vi "get db wheel info.vi"() -> ()   [LabVIEW 2016]
uses:
  <vilib>/addons/database/Connection.llb/DB Tools Open Connec (String).vi
  <vilib>/addons/database/Connection.llb/Conn Execute.vi
  <vilib>/addons/database/Recordset.llb/Rec Fetch Recordset Data (R).vi
  <vilib>/addons/database/Recordset.llb/Rec Destroy - Connection.vi
  <vilib>/Utility/file.llb/Write Delimited Spreadsheet (string).vi
  <vilib>/addons/database/NI_Database_API.lvlib
panel:
  out "size(s)":i32
  out "data":timestamp[](array[timestamp])
  out "date/time string 2":string
  out "date/time string":string
  out "sorted array":timestamp[](array[timestamp])
  out "element":string
  out "output array":string[][](array[string])
  out "Array 3":string[](array[string])
  out "Numeric":i32
  out "Array 4":string[](array[string])
  out "subarray":string[](array[string])
  out "Array 2":i16[](array[numeric])
  out "qa per group":dbl
  out "blanks per group":dbl
  out "unknown per group":dbl
  out "number of groups":dbl
  out "unknowns":i32
  out "qa number of":i32
  out "blanks number of":i32
  out "standards number of":i32
  out "x-y":dbl[](array[numeric])
  out "recordset data 2":variant[][](array[variant])
  out "concatenated string":string
  in  "wheel number":dbl=1.0
  out "error out 2":errorcluster
  in  "Ring":u16(ring)=1 items=["10Be"=1, "14C"=2, "26Al"=3, "36Cl"=5, "41Ca"=6, "129I"=7]
  out "Array":string[](array[string])
  out "error out":errorcluster
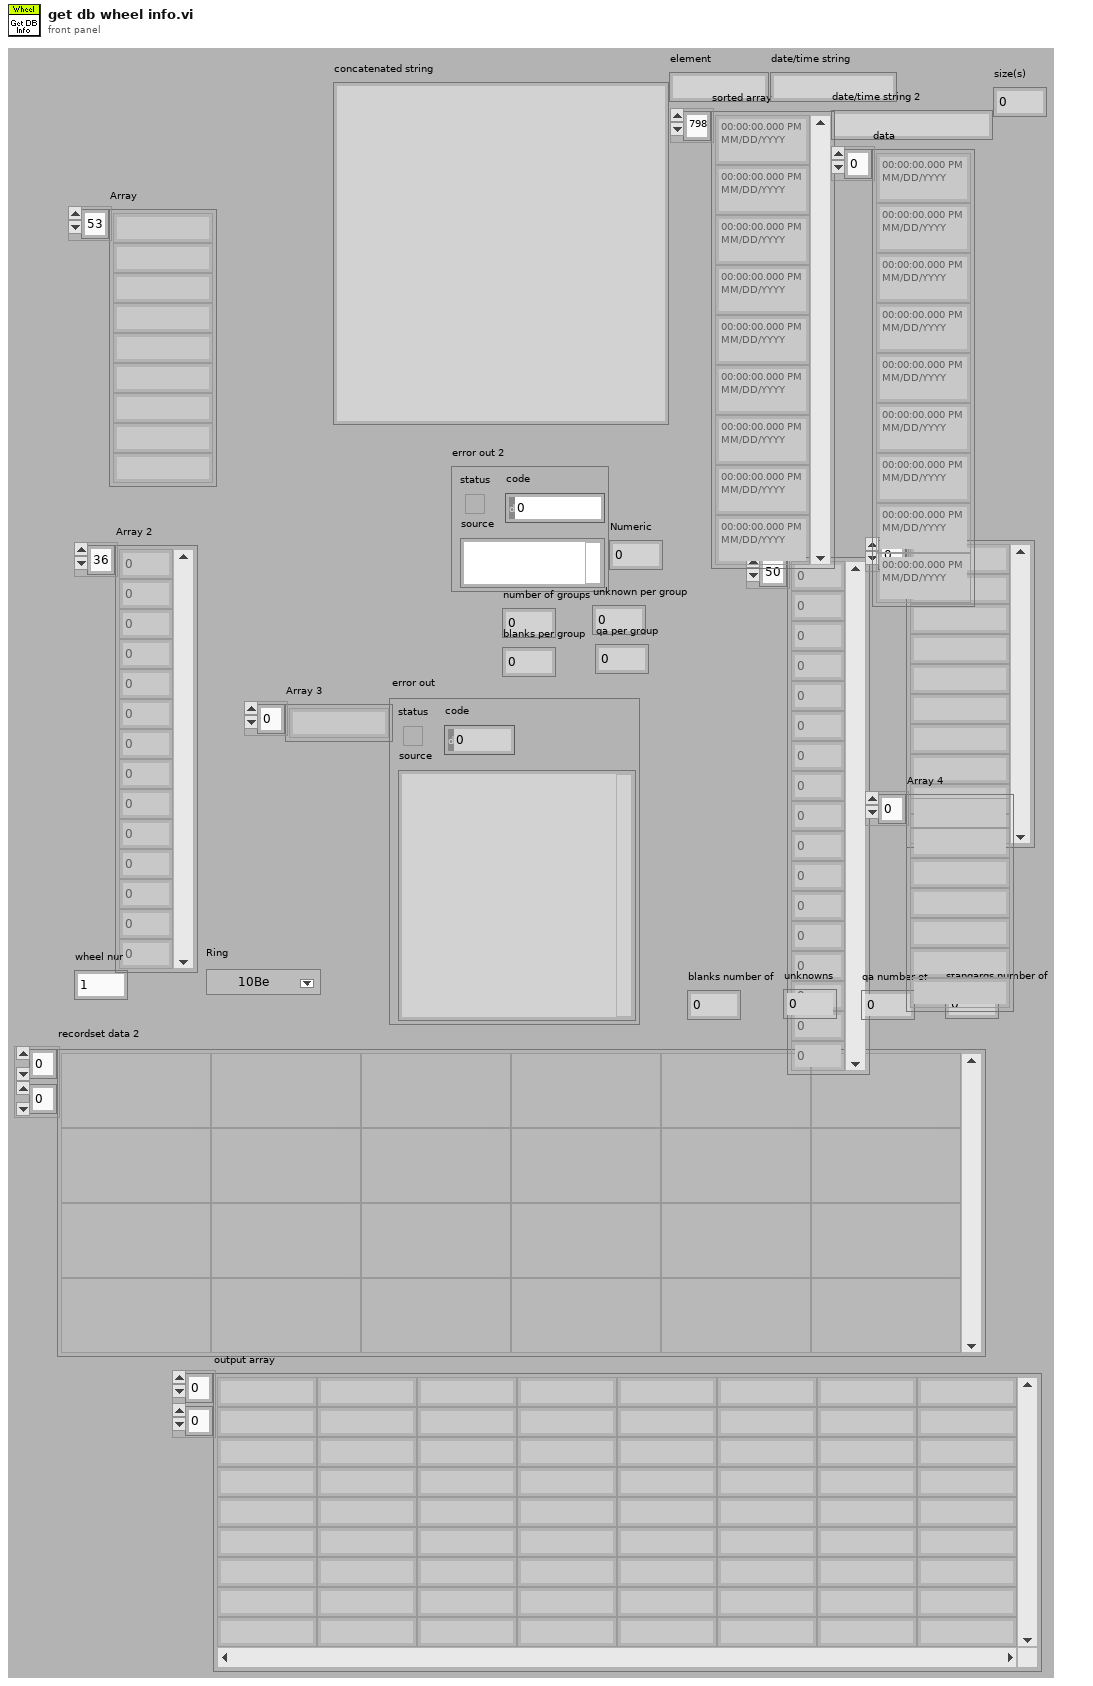
[diagram p1: front panel]
types:
  T1 = typedef "NI_Database_API.lvlib/Conn ObjectReference.ctl" = refnum<k1>
  T2 = typedef "NI_Database_API.lvlib/Rec ObjectReference.ctl" = refnum<k1>
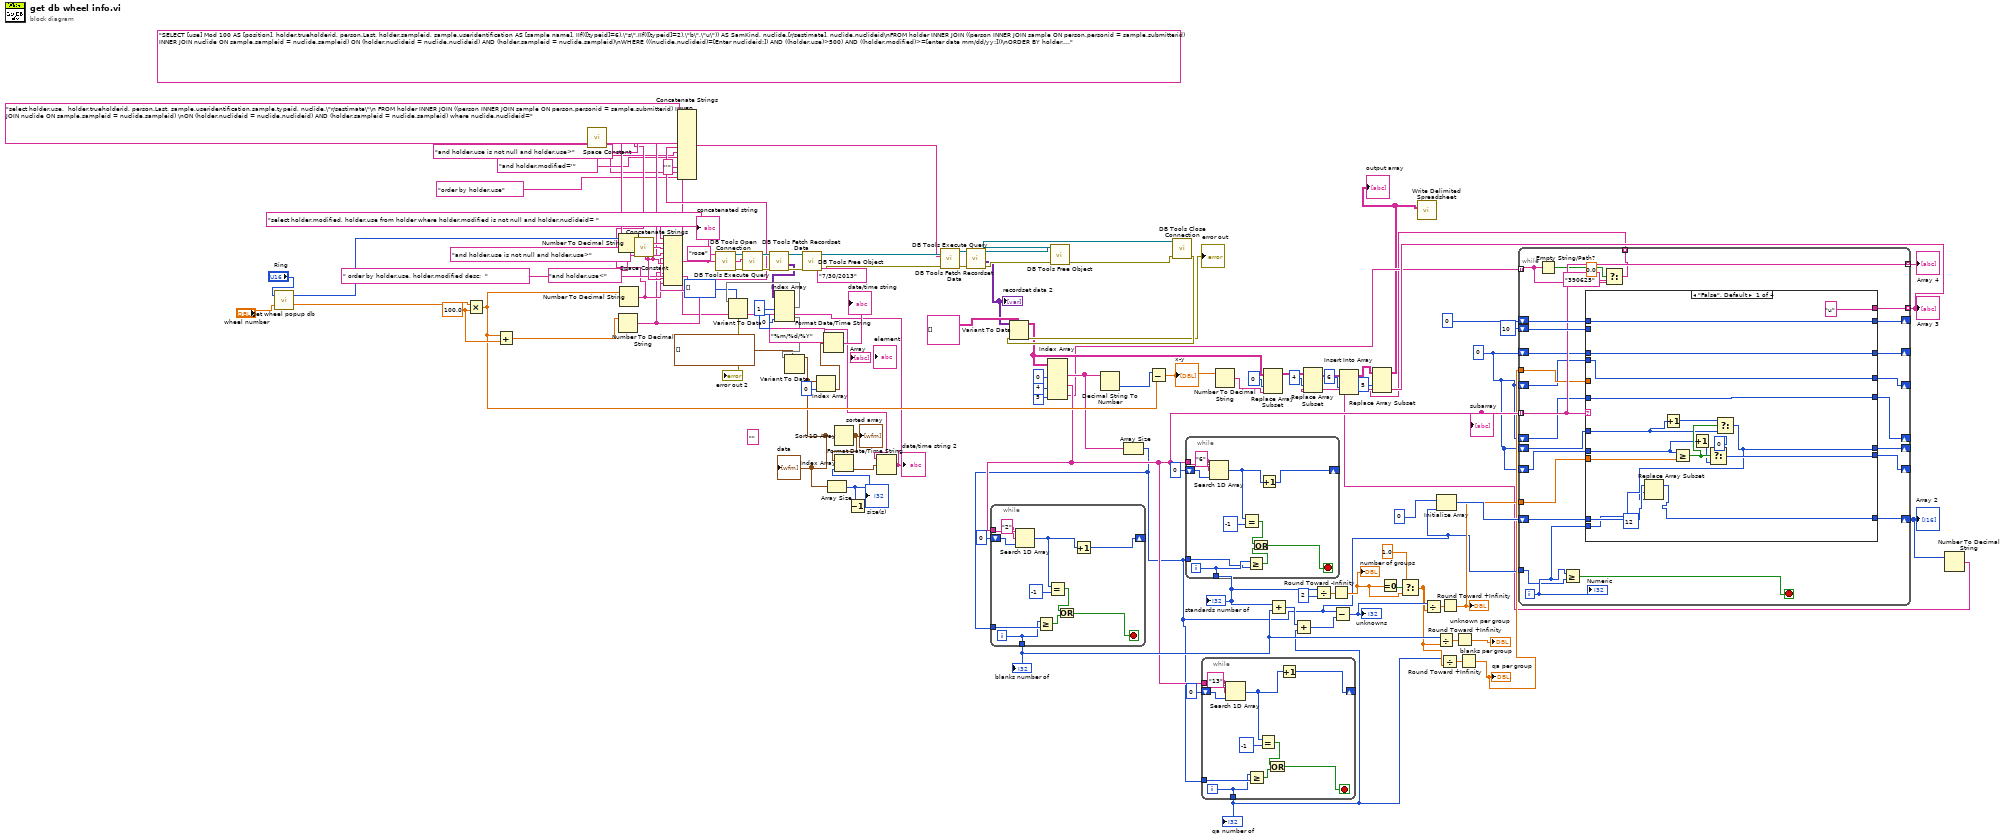
[diagram p0: block diagram]
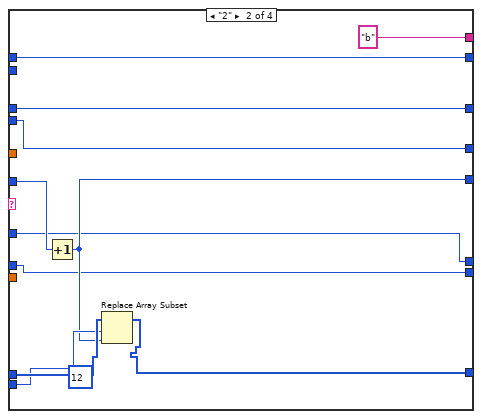
[diagram p2: hidden frame]
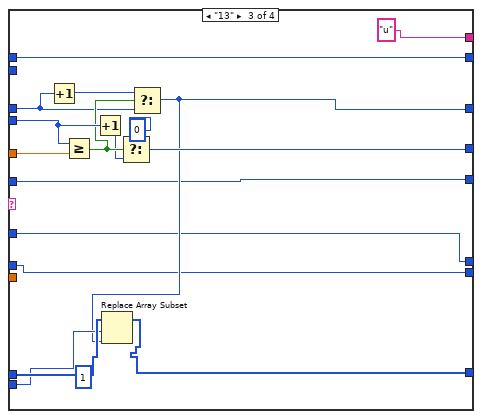
[diagram p3: hidden frame]
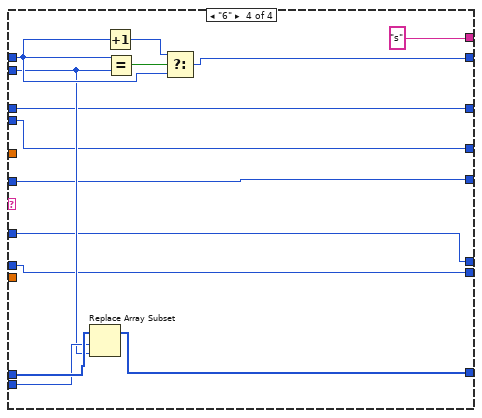
[diagram p4: hidden frame]
diagram:
  w6 = "%m/%d/%Y" ("time format string (%c)")
  (unwired) ""
  (unwired) "7/30/2013" ("element")
  w30 = i8 0 ("t")
  (unwired) "SELECT [use] Mod 100 AS [position], holder.trueholderid, person.Last, holder.sampleid, sample.useridentification AS [sample name], IIf(([typeid]=6),\"s\",IIf(([typeid]=2),\"b\",\"u\")) AS SamKind, nuclide.[r/sestimate], nuclide.nuclideid\nFROM holder INNER JOIN ((person INNER JOIN sample ON person.personid = sample.submitterid) INNER JOIN nuclide ON sample.sampleid = nuclide.sampleid) ON (holder.nuclideid = nuclide.nuclideid) AND (holder.sampleid = nuclide.sampleid)\nWHERE (((nuclide.nuclideid)=[Enter nuclideid:]) AND ((holder.use)>500) AND ((holder.modified)>=[enter date mm/dd/yy:]))\nORDER BY holder.use, [use] Mod 100" ("SQL query")
  w74 = "and holder.use<" ("SQL query")
  w90 = 100.0 ("y")
  n1 = call "get wheel popup db.vi"("wheel number"="wheel number", "Ring"="Ring") -> ("wheel number 2"=w91:dbl, "Ring 2"=w95:u16)
  n2 = Multiply(x=w91, y=w90) -> (x*y=w59:dbl)
  n3 = Add(x=w59, y=w90) -> (x+y=w89:dbl)
  n4 = call <vilib>:"Space Constant.vi"() -> ("String"=w69:string)
  n5 = Number To Decimal String(number=w89) -> (decimal integer string=w73:string)  [unwired: 1 in]
  n6 = Number To Decimal String(number=w95) -> (decimal integer string=w77:string)  [unwired: 1 in]
  n7 = Number To Decimal String(number=w59) -> (decimal integer string=w75:string)  [unwired: 1 in]
  n8 = call <vilib>:"Space Constant.vi"() -> ("String"=w88:string)
  n9 = Concatenate Strings("select holder.modified, holder.use from holder where holder.modified is not null and holder.nuclideid= " ("SQL query"), w77, w88, "and holder.use is not null and holder.use>" ("SQL query"), w75, w88, w74, w73, w88, " order by holder.use, holder.modified desc;  " ("SQL query")) -> (w94:string)
  "concatenated string" <- w94
  n10 = call-poly <vilib>:"DB Tools Open Connection.vi"("connection information"="rose") -> ("error out"=w104:errorcluster, "connection reference"=w105:T1)  [unwired: 7 in]
  n11 = call-poly <vilib>:"DB Tools Execute Query.vi"("error in (no error)"=w104, "SQL query"=w94, "connection reference"=w105) -> ("error out"=w108:errorcluster, "recordset reference"=w107:T2)  [unwired: 5 in]
  n12 = call-poly <vilib>:"DB Tools Fetch Recordset Data.vi"("error in (no error)"=w108, "recordset reference"=w107) -> ("error out"=w110:errorcluster, "recordset data"=w92:variant[][], "recordset reference out"=w109:T2)  [unwired: 3 in]
  n13 = Index Array(array=w92, index (col) #1=1 ("disabled index (col)"), index (col) #2=0 ("index (col)")) -> (element #1=w102:variant[], element #2=w99:variant[])  [unwired: 2 in]
  n14 = Variant To Data(type=i32[] [], Variant=w102) -> (error out=→"error out 2":errorcluster)  [unwired: 1 in, 1 out]
  n15 = Variant To Data(type=timestamp[] [], Variant=w99) -> (data=w9:timestamp[])  [unwired: 1 in, 1 out]
  "data" <- w9
  n16 = call-poly <vilib>:"DB Tools Free Object.vi"("error in (no error)"=w110, "recordset reference"=w109) -> ("error out"=w85:errorcluster, "connection reference"=w84:T1)  [unwired: 8 in]
  n17 = Index Array(array=w9, index=0) -> (element=w11:timestamp)
  n18 = Format Date/Time String(time format string (%c)=w6, seconds (now)=w11) -> (date/time string=→"date/time string":string)  [unwired: 1 in]
  n19 = Array Size(array=w9) -> (size(s)=w7:i32)
  "size(s)" <- w7
  n20 = Sort 1D Array(array=w9) -> (sorted array=w3:timestamp[])
  "sorted array" <- w3
  n21 = Decrement(x=w7) -> (x-1=w4:i32)
  n22 = Index Array(array=w3, index=w4) -> (element=w8:timestamp)
  n23 = Format Date/Time String(time format string (%c)=w6, seconds (now)=w8) -> (date/time string=w2:string)  [unwired: 1 in]
  "date/time string 2" <- w2
  n24 = Concatenate Strings("select holder.use,  holder.trueholderid, person.Last, sample.useridentification,sample.typeid, nuclide.\"r/sestimate\"\n FROM holder INNER JOIN ((person INNER JOIN sample ON person.personid = sample.submitterid) INNER JOIN nuclide ON sample.sampleid = nuclide.sampleid) \nON (holder.nuclideid = nuclide.nuclideid) AND (holder.sampleid = nuclide.sampleid) where nuclide.nuclideid=" ("SQL query"), w77, w69, "and holder.use is not null and holder.use>" ("SQL query"), w75, w69, w74, w73, w69, "and holder.modified='" ("string"), w2, "'" ("string"), w69, "order by holder.use" ("string")) -> (w72:string)
  n25 = call-poly <vilib>:"DB Tools Execute Query.vi"("error in (no error)"=w85, "SQL query"=w72, "connection reference"=w84) -> ("error out"=w79:errorcluster, "recordset reference"=w86:T2)  [unwired: 5 in]
  n26 = call-poly <vilib>:"DB Tools Fetch Recordset Data.vi"("error in (no error)"=w79, "recordset reference"=w86) -> ("error out"=w83:errorcluster, "recordset data"=w66:variant[][], "recordset reference out"=w82:T2)  [unwired: 3 in]
  "recordset data 2" <- w66
  n27 = call-poly <vilib>:"DB Tools Free Object.vi"("error in (no error)"=w83, "recordset reference"=w82) -> ("error out"=w80:errorcluster, "connection reference"=w81:T1)  [unwired: 8 in]
  n28 = call <vilib>:"DB Tools Close Connection.vi"("error in (no error)"=w80, "connection reference"=w81) -> ("error out"=w65:errorcluster)  [unwired: 5 in]
  n29 = Variant To Data(error in=w65, type=string[][] [], Variant=w66) -> (data=w28:string[][], error out=→"error out":errorcluster)
  n30 = Index Array(array=w28, index (col) #1=0 ("disabled index (col)"), index (col) #2=4 ("index (col)"), index (col) #3=5 ("index (col)")) -> (element #1=w58:string[], element #2=w38:string[], element #3=w15:string[])  [unwired: 3 in]
  "subarray" <- w38
  n31 = Decimal String To Number(string=w58) -> (number=w60:i32[])  [unwired: 2 in, 1 out]
  n32 = Array Size(array=w58) -> (size(s)=w26:i32)
  n33 = while {
    tunnel: w38 -> [w121]
    shift-right: [w111] -> _
    shift-left: 0 ("index of element") -> [w119]
    tunnel: w26 -> [w116]
    tunnel: [w113] -> w44
    i -> [w113]
    stop <- w114 stop-if-true
    n34 = Search 1D Array(1D array=w121, element="2", start index (0)=w119) -> (index of element=w112:i32)
    n35 = Greater Or Equal?(x=w113, y=w116) -> (x >= y?=w115:bool)
    n36 = Equal?(x=w112, y=-1) -> (x = y?=w117:bool)
    n37 = Or(x=w117, y=w115) -> (x .or. y?=w114:bool)
    n38 = Increment(x=w112) -> (x+1=w111:i32)
  }
  "blanks number of" <- w44
  n39 = Subtract(x=w60, y=w59) -> (x-y=w29:dbl[])
  "x-y" <- w29
  n40 = while {
    tunnel: w38 -> [w132]
    shift-right: [w125] -> _
    shift-left: 0 ("index of element") -> [w130]
    tunnel: w26 -> [w122]
    tunnel: [w123] -> w52
    i -> [w123]
    stop <- w127 stop-if-true
    n41 = Search 1D Array(1D array=w132, element="6", start index (0)=w130) -> (index of element=w126:i32)
    n42 = Equal?(x=w126, y=-1) -> (x = y?=w128:bool)
    n43 = Greater Or Equal?(x=w123, y=w122) -> (x >= y?=w124:bool)
    n44 = Or(x=w128, y=w124) -> (x .or. y?=w127:bool)
    n45 = Increment(x=w126) -> (x+1=w125:i32)
  }
  "standards number of" <- w52
  n46 = while {
    tunnel: w38 -> [w143]
    shift-right: [w133] -> _
    shift-left: 0 ("index of element") -> [w141]
    tunnel: w26 -> [w138]
    tunnel: [w135] -> w39
    i -> [w135]
    stop <- w136 stop-if-true
    n47 = Search 1D Array(1D array=w143, element="13", start index (0)=w141) -> (index of element=w134:i32)
    n48 = Greater Or Equal?(x=w135, y=w138) -> (x >= y?=w137:bool)
    n49 = Equal?(x=w134, y=-1) -> (x = y?=w139:bool)
    n50 = Or(x=w139, y=w137) -> (x .or. y?=w136:bool)
    n51 = Increment(x=w134) -> (x+1=w133:i32)
  }
  "qa number of" <- w39
  n52 = Number To Decimal String(number=w29) -> (decimal integer string=w27:string[])  [unwired: 1 in]
  n53 = Replace Array Subset(array=w28, new element=w27, index (col)=0 ("disabled index (col)")) -> (w25:string[][])  [unwired: 1 in]
  n54 = Add(x=w52, y=w44) -> (x+y=w54:i32)
  n55 = Add(x=w54, y=w39) -> (x+y=w53:i32)
  n56 = Divide(x=w52, y=2) -> (x/y=w50:dbl)
  n57 = Round Toward -Infinity(1:w50) -> (0:w47:dbl)
  "number of groups" <- w47
  n58 = Subtract(x=w26, y=w53) -> (x-y=w46:i32)
  "unknowns" <- w46
  n59 = Equal To 0?(x=w47) -> (x = 0?=w49:bool)
  n60 = Select(t=1.0, s=w49, f=w47) -> (s? t:f=w43:dbl)
  n61 = Divide(x=w46, y=w43) -> (x/y=w45:dbl)
  n62 = Divide(x=w44, y=w43) -> (x/y=w41:dbl)
  n63 = Initialize Array(i16 0 ("t"), w26) -> (w37:i16[])
  n64 = Divide(x=w39, y=w43) -> (x/y=w42:dbl)
  n65 = Round Toward +Infinity(x=w45) -> (ceil(x): smallest int >= x=w31:dbl)
  "unknown per group" <- w31
  n66 = Round Toward +Infinity(x=w41) -> (ceil(x): smallest int >= x=→"blanks per group":dbl)
  n67 = Round Toward +Infinity(x=w42) -> (ceil(x): smallest int >= x=w32:dbl)
  "qa per group" <- w32
  n68 = while {
    tunnel: w26 -> [w161]
    tunnel: w38 -> [w163] mode=indexing
    shift-right: [w164] -> w22
    shift-left: w37 -> [w168]
    shift-right: [w165] -> _
    shift-left: i8 0 ("t") -> [w167]
    shift-left: i8 10 ("t") -> [w166]
    tunnel: [w163] -> w33 mode=indexing
    tunnel: w32 -> [w160]
    shift-right: [w156] -> _
    shift-left: w30 -> [w159]
    shift-right: [w157] -> _
    shift-left: w30 -> [w158]
    shift-right: [w154] -> _
    shift-left: w30 -> [w155]
    tunnel: w31 -> [w153]
    shift-right: [w151] -> _
    shift-left: w30 -> [w152]
    shift-right: [w149] -> _
    shift-left: w30 -> [w150]
    tunnel: [w148] -> w24 mode=indexing
    tunnel: w15 -> [w146] mode=indexing
    tunnel: [w144] -> w12 mode=indexing
    i -> [w162]
    stop <- w169 stop-if-true
    (unwired) 0.0 ("t")
    n69 = Empty String/Path?(string/path=w146) -> (empty?=w147:bool)
    n70 = Greater Or Equal?(x=w162, y=w161) -> (x >= y?=w169:bool)
    n71 = case shown="\"False\", Default" w163 {
      tunnel: w168 -> [w185 w196 w213 w226]
      tunnel: w162 -> [w184 w195 w212 w225]
      tunnel: w167 -> [w186 w197 w214 w224]
      tunnel: w166 -> [_ _ _ w221]
      tunnel: [w186 w197 w214 w222] -> w165
      tunnel: [w183 w194 w211 w223] -> w164
      tunnel: w160 -> [_ _ w210 _]
      tunnel: w159 -> [w181 w192 w202 w219]
      tunnel: w158 -> [w182 w193 w209 w220]
      tunnel: [w182 w193 w208 w220] -> w157
      tunnel: [w181 w192 w206 w219] -> w156
      tunnel: w155 -> [w180 w191 w201 w218]
      tunnel: [w180 w190 w201 w218] -> w154
      tunnel: w153 -> [w176 _ _ _]
      tunnel: w152 -> [w175 w189 w200 w217]
      tunnel: [w174 w189 w200 w217] -> w151
      tunnel: w150 -> [w173 w188 w199 w216]
      tunnel: [w172 w188 w199 w216] -> w149
      tunnel: ["u" ("element") "b" ("element") "u" ("element") "s" ("element")] -> w148
      frame "False", Default {
        (unwired) i16 12 ("new element/subarray")
        n72 = Increment(x=w173) -> (x+1=w177:i8)
        n73 = Greater Or Equal?(x=w175, y=w176) -> (x >= y?=w179:bool)
        n74 = Increment(x=w175) -> (x+1=w178:i8)
        n75 = Select(t=i8 0 ("f"), s=w179, f=w178) -> (s? t:f=w174:i8)
        n76 = Select(t=w177, s=w179, f=w173) -> (s? t:f=w172:i8)
        n77 = Replace Array Subset(array=w185, new element=w172, index=w184) -> (w183:i16[])
      }
      frame "2" {
        (unwired) i16 12 ("new element/subarray")
        n78 = Increment(x=w191) -> (x+1=w190:i8)
        n79 = Replace Array Subset(array=w196, new element=w190, index=w195) -> (w194:i16[])
      }
      frame "13" {
        (unwired) i16 1 ("new element/subarray")
        n80 = Increment(x=w202) -> (x+1=w203:i8)
        n81 = Greater Or Equal?(x=w209, y=w210) -> (x >= y?=w207:bool)
        n82 = Increment(x=w209) -> (x+1=w204:i8)
        n83 = Select(t=i8 0 ("f"), s=w207, f=w204) -> (s? t:f=w208:i8)
        n84 = Select(t=w203, s=w207, f=w202) -> (s? t:f=w206:i8)
        n85 = Replace Array Subset(array=w213, new element=w206, index=w212) -> (w211:i16[])
      }
      frame "6" {
        n86 = Replace Array Subset(array=w226, new element=w221, index=w225) -> (w223:i16[])
        n87 = Increment(x=w224) -> (x+1=w227:i8)
        n88 = Equal?(x=w224, y=w221) -> (x = y?=w228:bool)
        n89 = Select(t=w227, s=w228, f=w224) -> (s? t:f=w222:i8)
      }
    }
    n90 = Select(t="390625", s=w147, f=w146) -> (s? t:f=w144:string)
    "Numeric" <- w162
  }
  "Array 2" <- w22
  "Array 4" <- w33
  "Array 3" <- w24
  n91 = Replace Array Subset(array=w25, new element=w24, index (col)=4 ("disabled index (col)")) -> (w23:string[][])  [unwired: 1 in]
  n92 = Number To Decimal String(number=w22) -> (decimal integer string=w21:string[])  [unwired: 1 in]
  n93 = Insert Into Array(array=w23, index (col)=6 ("disabled index (col)"), new element=w21) -> (w14:string[][])  [unwired: 1 in]
  n94 = Replace Array Subset(array=w14, new element=w12, index (col)=5 ("disabled index (col)")) -> (w1:string[][])  [unwired: 1 in]
  "output array" <- w1
  n95 = call-poly <vilib>:"Write Delimited Spreadsheet.vi"("2D data"=w1) -> ()  [unwired: 13 in, 2 out]
